vi "sweep_finished.vi"(8 "error in (no error)":errorcluster, 11 "DataCollectionDL090215 in":refnum<class "DataCollectionDL090215.lvclass">) -> (0 "error out":errorcluster, 3 "DataCollectionDL090215 out":refnum<class "DataCollectionDL090215.lvclass">)   [LabVIEW 2010, in "DataCollectionDL090215.lvclass"]
uses:
  DataCollectionDL090215.lvclass
  DataCollectionDL091104Scaffold/DataCollectionDL091104Scaffold/DataCollectionDL091104Scaffold.lvclass
  DataCollectionDL090215.lvclass/DataCollectionDL090215.ctl
  GenericDataCollection/GenericDataCollection/trigger_enum.ctl
  GenericDataCollection/GenericDataCollection/GenericDataCollection.lvclass
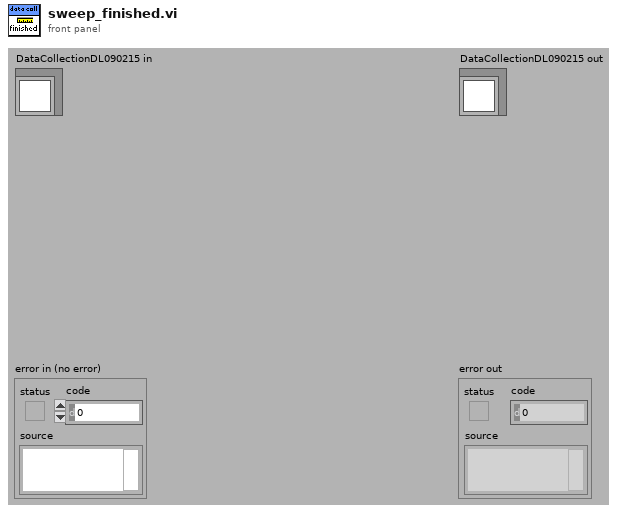
[diagram p1: front panel]
types:
  T1 = typedef "GenericDataCollection.lvclass/trigger_enum.ctl" = enum16{"NULL", "save", "reset"}
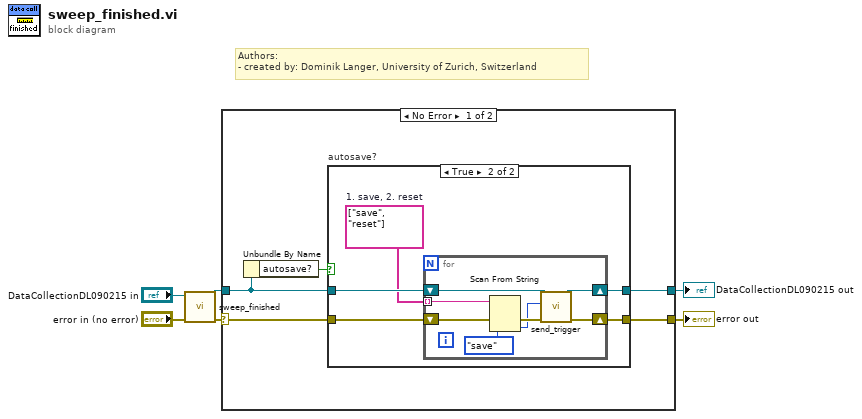
[diagram p0: block diagram]
diagram:
  # "Authors: \n- created by: Dominik Langer, University of Zurich, Switzerland"
  n1 = call-parent "sweep_finished.vi"("error in (no error)"="error in (no error)", "DataCollectionDL091104Scaffold in"="DataCollectionDL090215 in") -> ("error out"=w4:errorcluster, "DataCollectionDL091104Scaffold out"=w3:refnum<class "DataCollectionDL090215.lvclass">)  [unwired: 8 in]
  n2 = case shown="No Error" w4 {
    selector: w4 -> [w11 w28]
    tunnel: w3 -> [w10 w27]
    tunnel: [w8 w28] -> w2
    tunnel: [w7 w27] -> w1
    frame No Error {
      n3 = Unbundle By Name(w10) -> ("autosave?"=w9:bool)
      n4 = case "autosave?" shown="True" w9 {
        tunnel: w11 -> [w13 w17]
        tunnel: [w13 w16] -> w8
        tunnel: [w12 w15] -> w7
        tunnel: w10 -> [w12 w18]
        frame False {
        }
        frame True {
          w14 = string[] ["save", "reset"]  # 1. save, 2. reset
          n5 = for {
            tunnel: w14 -> [w20] mode=indexing
            shift-right: [w25] -> w16
            shift-left: w17 -> [w22]
            shift-right: [w24] -> w15
            shift-left: w18 -> [w26]
            n6 = Scan From String(input string=w20, error in=w22, default 1=trigger_enum."save" ("save")) -> (error out=w23:errorcluster, output 1=w19:T1)  [unwired: 2 in, 2 out]
            n7 = call-dynamic "send_trigger.vi"("error in (no error)"=w23, "trigger"=w19, "GenericDataCollection in"=w26) -> ("error out"=w25:errorcluster, "GenericDataCollection out"=w24:refnum<class "DataCollectionDL090215.lvclass">)  [unwired: 7 in]
          }
        }
      }
    }
    frame Error {
    }
  }
  "error out" <- w2
  "DataCollectionDL090215 out" <- w1
